vi "SetArmPosition.vi"   [LabVIEW 2015]
uses:
  Utilities/MotorPositionGlobals.vi
types:
  T1 = typedef "WPI_MotorControlDeviceRef.ctl" = cluster{"DeviceStatus":errorcluster, "Type":T2, "PWM":cluster{"PWM Channel":T3, "DeadBand":T4}, "CAN":cluster{"Device Number":u8, "Control Mode":T5, "Semaphore":T6, "Max Vout":dbl, "TalonSRX Control Mode":T7}, "Invert":bool}
  T2 = typedef "WPI_MotorControlType.ctl" = enum16{"PWM", "CAN", "CANTalonSRX"}
  T3 = typedef "FPGA_DIOPWMChannel.ctl" = enum8{"PWM 0", "PWM 1", "PWM 2", "PWM 3", "PWM 4", "PWM 5", "PWM 6", "PWM 7", "PWM 8", "PWM 9", "PWM MXP 0", "PWM MXP 1", "PWM MXP 2", "PWM MXP 3", "PWM MXP 4", "PWM MXP 5", "PWM MXP 6", "PWM MXP 7", "PWM MXP 8", "PWM MXP 9", "Invalid"}
  T4 = typedef "WPI_PWMDeadband.ctl" = cluster{"Name":string, "maxPositivePwm":i32, "minPositivePwm":i32, "centerPwm":i32, "maxNegativePwm":i32, "minNegativePwm":i32, "angularRange":u16}
  T5 = typedef "WPI_CANJaguar_ControlMode.ctl" = enum8{"Percent VBus", "Current", "Speed", "Position", "Voltage"}
  T6 = typedef "Semaphore RefNum" = refnum<k1>
  T7 = typedef "WPI_CANTalonSRX_APIControlMode.ctl" = enum8{"Percent VBus", "Speed", "Position", "Slave", "Unchanged / Invalid", "Voltage Compensation", "Current", "Motion Profile"}
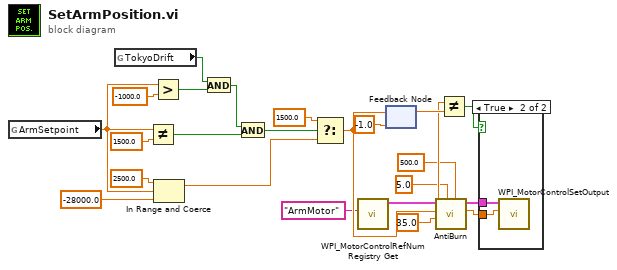
[diagram p0: block diagram]
diagram:
  n1 = global read "MotorPositionGlobals.vi" "ArmSetpoint"() -> (w12:dbl)
  n2 = global read "MotorPositionGlobals.vi" "TokyoDrift"() -> (w13:bool)
  n3 = Not Equal?(x=w12, y=1500.0) -> (x != y?=w18:bool)
  n4 = Greater?(x=w12, y=-1000.0) -> (0:w10:bool)
  n5 = In Range and Coerce(upper limit=2500.0, x=w12, lower limit=-28000.0) -> (coerced(x)=w20:dbl)  [unwired: 1 out]
  n6 = And(x=w13, y=w10) -> (x .and. y?=w9:bool)
  n7 = And(x=w9, y=w18) -> (x .and. y?=w17:bool)
  n8 = Select(t=1500.0, s=w17, f=w20) -> (s? t:f=w8:dbl)
  n9 = call <vilib>:"WPI_MotorControlRefNum Registry Get.vi"("refnum name"="ArmMotor") -> ("MotorControlDevRef"=w1:T1)  [unwired: 9 in, 1 out]
  n10 = feedback-in #1(w8) -> ()
  n11 = feedback #1(-1.0 ("upper limit")) -> (w16:dbl)
  n12 = call "AntiBurn.vi"("AllowedEncoderError"=500.0, "AllowedTimeDeviation"=5.0, "MaxCurrent"=35.0, "MotorSetpoint"=w8, "CAN Talon SRX Ref"=w1) -> ("MotorSetpointOut"=w7:dbl, "MotorControlDevRef"=w6:T1)  [unwired: 3 in, 2 out]
  n13 = Not Equal?(x=w8, y=w16) -> (x != y?=w14:bool)
  n14 = case shown="True" w14 {
    tunnel: w6 -> [_ w25]
    tunnel: w7 -> [_ w24]
    frame False {
    }
    frame True {
      n15 = call <vilib>:"WPI_MotorControlSetOutput.vi"("Output"=w24, "MotorControlDevRef"=w25) -> ()  [unwired: 7 in, 3 out]
    }
  }
